vi "getInputsOutputsFolder.vi"(8 "error in (no error)":errorcluster, 11 "IDevice in":refnum<class "IDevice.lvclass">) -> (0 "error out":errorcluster, 2 "IFolder out":refnum<class "IFolder.lvclass">, 3 "IDevice out":refnum<class "IDevice.lvclass">)   [LabVIEW 2022 SP3, in "openDAQ.lvlib" / "IBaseObject.lvlib" / "IPropertyObject.lvlib" / "IComponent.lvlib" / "IFolder.lvlib" / "IDevice.lvlib" / "IDevice.lvclass"]
uses:
  <instrlib>/openDAQ/Public/Classes/IDevice/IDevice.lvclass
  <instrlib>/openDAQ/Public/Classes/IDevice/IDevice.lvclass/IDevice.ctl
  <instrlib>/openDAQ/Binaries/Windows/x86/copendaq32.dll
  <instrlib>/openDAQ/Public/Classes/IFolder/IFolder.lvclass
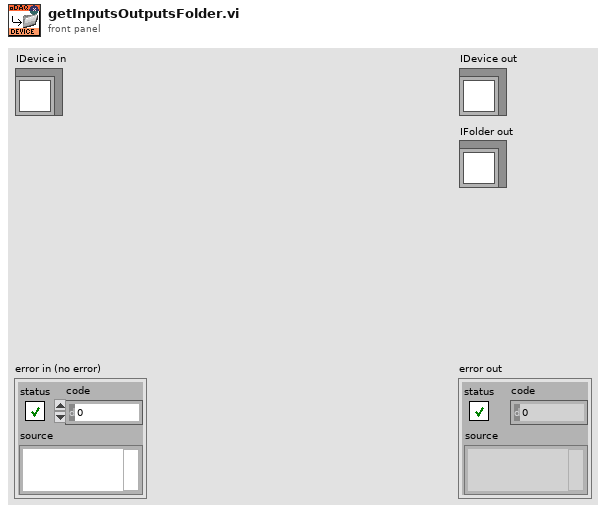
[diagram p1: front panel]
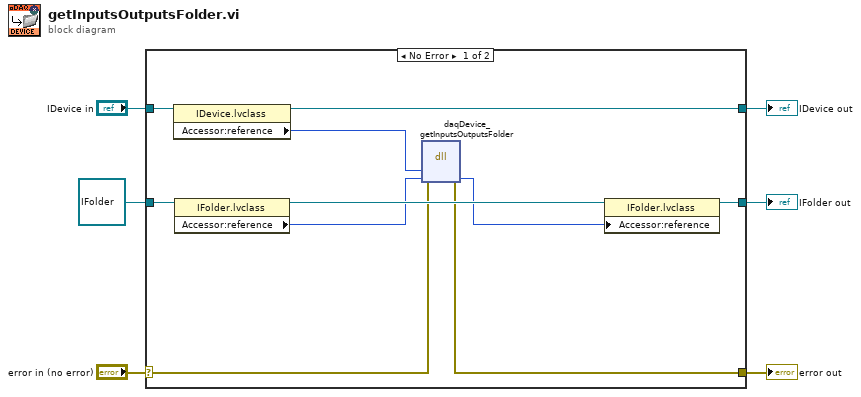
[diagram p0: block diagram]
diagram:
  n1 = case shown="No Error" "error in (no error)" {
    selector: "error in (no error)" -> [w12 w19]
    tunnel: [w11 w19] -> w5
    tunnel: [w10 w18] -> w3
    tunnel: "IDevice in" -> [w14 w18]
    tunnel: refnum<class "IFolder.lvclass"> refnum ("openDAQ.lvlib:IBaseObject.lvlib:IPropertyObject.lvlib:IComponent.lvlib:IFolder.lvlib:IFolder.lvclass") -> [w9 w17]
    tunnel: [w7 w17] -> w1
    frame No Error {
      n2 = property class="IDevice.lvclass"(reference=w14) -> (reference out=w10:refnum<class "IDevice.lvclass">, "Accessor:reference"=w13:i64)  [unwired: 1 in, 1 out]
      n3 = property class="IFolder.lvclass"(reference=w9) -> (reference out=w16:refnum<class "IFolder.lvclass">, "Accessor:reference"=w8:i64)  [unwired: 1 in, 1 out]
      n4 = dll-call lib="C:/Program Files (x86)/National Instruments/LabVIEW 2022/instr.lib/openDAQ/Binaries/Windows/x86/copendaq*.*" fn="daqDevice_getInputsOutputsFolder"(error in=w12, "device"=w13, "folder"=w8) -> (error out=w11:errorcluster, "folder"=w15:i64)  [unwired: 4 in, 1 out]
      n5 = property class="IFolder.lvclass"(reference=w16, "Accessor:reference"=w15) -> (reference out=w7:refnum<class "IFolder.lvclass">)  [unwired: 1 in, 1 out]
    }
    frame Error {
    }
  }
  "error out" <- w5
  "IDevice out" <- w3
  "IFolder out" <- w1
